vi "replaceXMLValue.vi"(8 "error in (no error)":errorcluster, 9 "value":string, 10 "replace in":string, 11 "NativeXML in":refnum<class "NativeXML.lvclass">) -> (0 "error out":errorcluster, 3 "NativeXML out":refnum<class "NativeXML.lvclass">)   [LabVIEW 2011, in "Tools.lvlib" / "xml.lvlib" / "NativeXML.lvclass"]
uses:
  NativeXML.lvclass
  NativeXML.lvclass/NativeXML.ctl
  <vilib>/xml/Close Reference(Node).vi
  Program Files/National Instruments/LabVIEW 2011/resource/objmgr/DOMUserDefRef.rc
  <vilib>/xml/NI_XML.lvlib
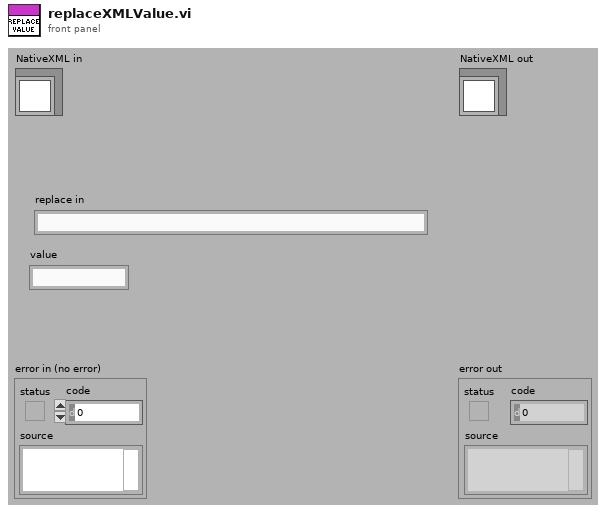
[diagram p1: front panel]
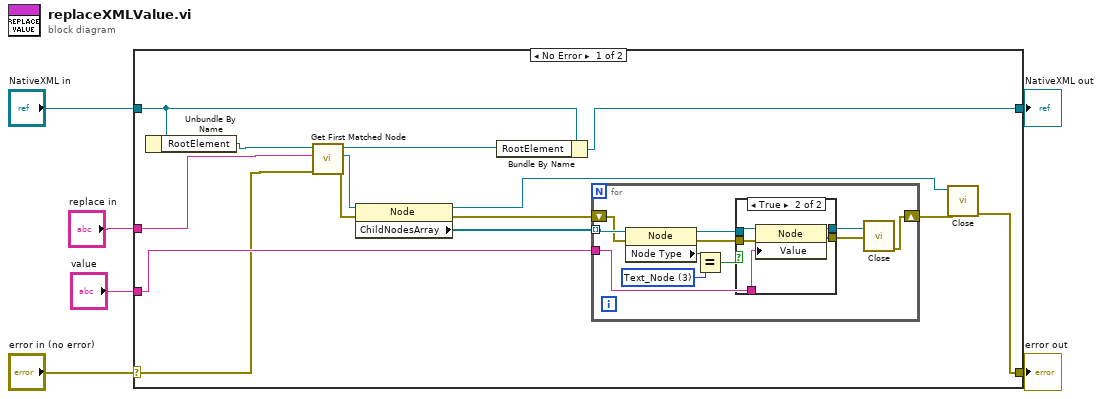
[diagram p0: block diagram]
diagram:
  n1 = case shown="No Error" "error in (no error)" {
    selector: "error in (no error)" -> [w15 w40]
    tunnel: [w7 w40] -> w5
    tunnel: [w19 w39] -> w3
    tunnel: "NativeXML in" -> [w20 w39]
    tunnel: "replace in" -> [w14 _]
    tunnel: "value" -> [w18 _]
    frame No Error {
      n2 = Unbundle By Name(w20) -> ("RootElement"=w17:refnum<k20>)
      n3 = call <vilib>:"Get First Matched Node.vi"("error in (no error)"=w15, "XPath expression"=w14, "node in"=w17) -> ("error out"=w10:errorcluster, "node result"=w13:refnum<k20>, "node out"=w16:refnum<k20>)  [unwired: 6 in]
      n4 = property class="Node"(reference=w13, error in=w10) -> (reference out=w8:refnum<k20>, error out=w11:errorcluster, "ChildNodesArray"=w12:refnum<k20>[])
      n5 = Bundle By Name(cluster=w20, "RootElement"=w16) -> (w19:refnum<class "NativeXML.lvclass">)
      n6 = for {
        tunnel: w18 -> [w21]
        tunnel: w12 -> [w26] mode=indexing
        shift-right: [w31] -> w9
        shift-left: w11 -> [w25]
        w27 = 3 items=["Element_Node"=1, "Attribute_Node"=2, "Text_Node"=3, "CDATASection_Node"=4, "EntityReference_Node"=5, "Entity_Node"=6, "ProcessingInstruction_Node"=7, "Comment_Node"=8, "Document_Node"=9, "DocumentType_Node"=10, "DocumentFragment_Node"=11, "Notation_Node"=12] ("Node Type")
        n7 = property class="Node"(reference=w26, error in=w25) -> (reference out=w24:refnum<k20>, error out=w23:errorcluster, "Node Type"=w28:i32)
        n8 = Equal?(x=w28, y=w27) -> (x = y?=w22:bool)
        n9 = case shown="True" w22 {
          tunnel: [w33 w38] -> w30
          tunnel: [w32 w37] -> w29
          tunnel: w24 -> [w33 w35]
          tunnel: w23 -> [w32 w34]
          tunnel: w21 -> [_ w36]
          frame False {
          }
          frame True {
            n10 = property class="Node"(reference=w35, error in=w34, "Value"=w36) -> (reference out=w38:refnum<k20>, error out=w37:errorcluster)
          }
        }
        n11 = call-poly <vilib>:"Close.vi"("error in (no error)"=w29, "node"=w30) -> ("error out"=w31:errorcluster)  [unwired: 7 in]
      }
      n12 = call-poly <vilib>:"Close.vi"("error in (no error)"=w9, "node"=w8) -> ("error out"=w7:errorcluster)  [unwired: 7 in]
    }
    frame Error {
    }
  }
  "error out" <- w5
  "NativeXML out" <- w3
